vi "NI VeriStand - Open Model.vi"(7 "Target":string, 8 "error in (no error)":errorcluster, 10 "Gateway IP Address (\"\": localhost)":string, 11 "Model Name":string) -> (0 "error out":errorcluster, 3 "Model":T1)   [LabVIEW 2020, in "NI_VS Model ExecutionAPI.lvlib"]
doc: "Opens a reference to a model. You must open a reference before using any other VIs on this palette."
uses:
  <vilib>/NI VeriStand/Execution/Model/NI_VS Model ExecutionAPI.lvlib
  <vilib>/NI VeriStand/Execution/Model/ModelAPI.ctl
  NationalInstruments.VeriStand.ClientAPI
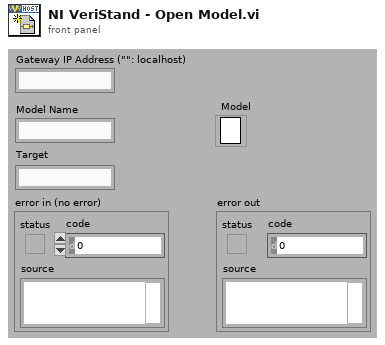
[diagram p1: front panel]
types:
  T1 = typedef "NI_VS Model ExecutionAPI.lvlib/ModelAPI.ctl" = refnum<k24>
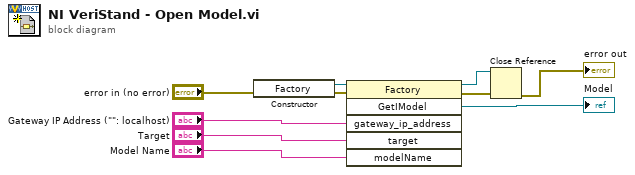
[diagram p0: block diagram]
diagram:
  n1 = constructor class="Factory"(error in="error in (no error)") -> (reference out=w9:refnum<k24>, error out=w10:errorcluster)  [unwired: 2 in, 1 out]
  n2 = invoke class="Factory" method="GetIModel"(reference=w9, error in=w10, "gateway_ip_address"="Gateway IP Address (\"\": localhost)", "target"="Target", "modelName"="Model Name") -> (reference out=w7:refnum<k24>, error out=w8:errorcluster, "GetIModel"=→"Model":refnum<k24>)  [unwired: 1 in, 3 out]
  n3 = Close Reference(reference=w7, error in (no error)=w8) -> (error out=→"error out":errorcluster)
